vi "Handle 1d Control Error.vi"(8 "Error In":errorcluster, 10 "TBL1D Refnum":refnum<vi>, 11 "Label":refnum<vi>) -> ()   [LabVIEW 2011]
uses:
  Tables/XCPCCP TBL1D.xctl
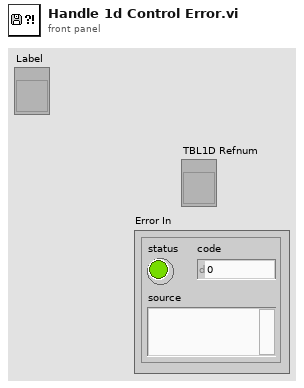
[diagram p1: front panel]
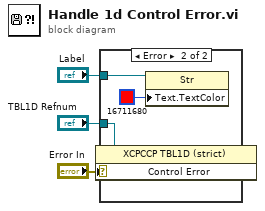
[diagram p0: block diagram]
diagram:
  n1 = case shown="Error" "Error In" {
    selector: "Error In" -> [_ w4]
    tunnel: "Label" -> [_ w7]
    tunnel: "TBL1D Refnum" -> [_ w5]
    frame No Error {
    }
    frame Error {
      n2 = property class="XCPCCP TBL1D (strict)"(reference=w5, "Control Error"=w4) -> ()  [unwired: 1 in, 2 out]
      n3 = property class="Str"(reference=w7, "Text.TextColor"=u32 16711680) -> ()  [unwired: 1 in, 2 out]
    }
  }
